vi "Filter-CF,BW to Flo, Fhi.vi"(8 "BW":dbl, 10 "CF (kHz)":dbl, 11 "BWUnits":T1) -> (0 "Fmin":dbl, 2 "Fmax":dbl)   [LabVIEW 2020]
uses:
  Filter-Bandwidth Units.ctl
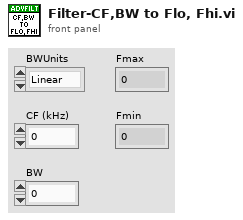
[diagram p1: front panel]
types:
  T1 = typedef "Filter-Bandwidth Units.ctl" = enum16{"Linear", "Octaves", "Min-Max"}
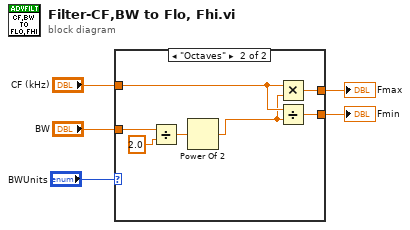
[diagram p0: block diagram]
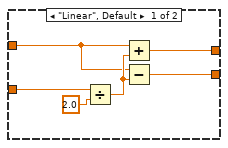
[diagram p2: hidden frame]
diagram:
  n1 = case shown="\"Octaves\"" "BWUnits" {
    tunnel: [w7 w15] -> w2
    tunnel: "CF (kHz)" -> [w9 w17]
    tunnel: [w6 w14] -> w1
    tunnel: "BW" -> [w8 w16]
    frame "Linear", Default {
      n2 = Divide(x=w8, y=2.0) -> (x/y=w11:dbl)
      n3 = Add(x=w9, y=w11) -> (x+y=w7:dbl)
      n4 = Subtract(x=w9, y=w11) -> (x-y=w6:dbl)
    }
    frame "Octaves" {
      n5 = Divide(x=w16, y=2.0) -> (x/y=w13:dbl)
      n6 = Power Of 2(x=w13) -> (2^x=w12:dbl)
      n7 = Multiply(x=w17, y=w12) -> (x*y=w15:dbl)
      n8 = Divide(x=w17, y=w12) -> (x/y=w14:dbl)
    }
  }
  "Fmin" <- w1
  "Fmax" <- w2
